vi "콜라 자판기.vi"() -> ()   [LabVIEW 2018]
panel:
  out "링":u16(ring)
  in  "종료":bool
  in  "반환":bool
  in  "구매":bool
  out "투입 금액":dbl
  in  "동전":cluster{bool, bool, bool, bool}
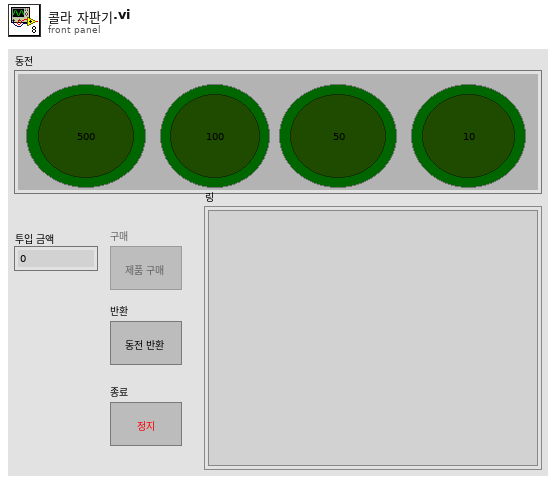
[diagram p1: front panel]
types:
  T1 = enum8{"Enabled", "Disabled", "Disabled and Grayed Out"}
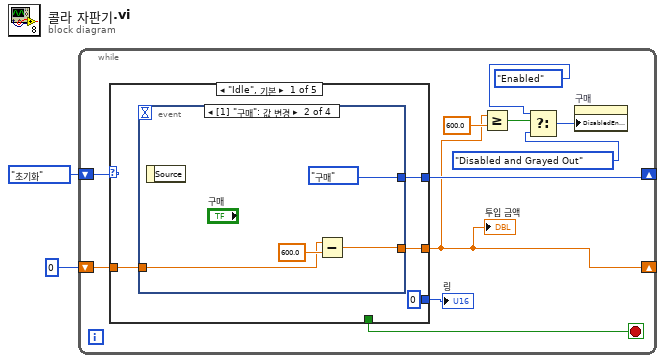
[diagram p0: block diagram]
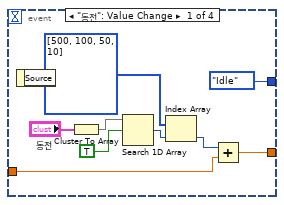
[diagram p2: hidden frame]
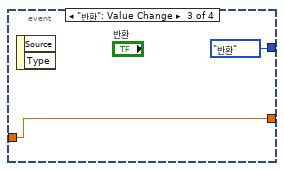
[diagram p3: hidden frame]
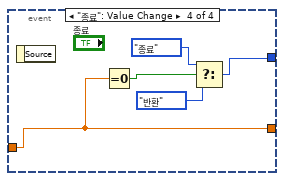
[diagram p4: hidden frame]
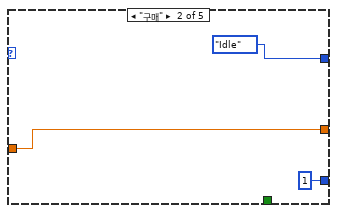
[diagram p5: hidden frame]
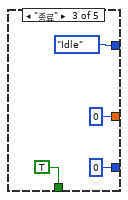
[diagram p6: hidden frame]
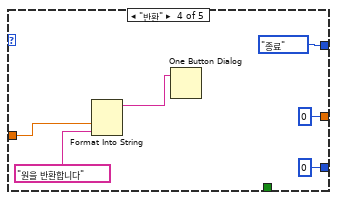
[diagram p7: hidden frame]
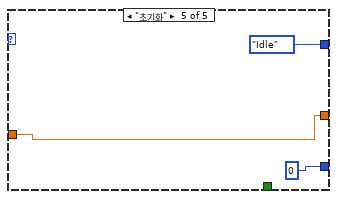
[diagram p8: hidden frame]
diagram:
  n1 = while {
    shift-right: [w12] -> _
    shift-left: enum16{"Idle", "초기화", "종료", "구매", "반환"}."초기화" ("열거형") -> [w13]
    shift-right: [w9] -> _
    shift-left: 0 -> [w11]
    stop <- w3 stop-if-true
    n2 = case shown="\"Idle\", 기본" w13 {
      tunnel: [w17 enum16{"Idle", "초기화", "종료", "구매", "반환"}."Idle" ("열거형") enum16{"Idle", "초기화", "종료", "구매", "반환"}."Idle" ("열거형") enum16{"Idle", "초기화", "종료", "구매", "반환"}."종료" ("열거형") enum16{"Idle", "초기화", "종료", "구매", "반환"}."Idle" ("열거형")] -> w12
      tunnel: [w16 w38 0 0 w53] -> w9
      tunnel: w11 -> [w15 w38 _ w47 w53]
      tunnel: [u16 0 ("링") u16 1 ("링") u16 0 ("링") u16 0 ("링") u16 0 ("링")] -> w4
      tunnel: [_ _ TRUE _ _] -> w3
      frame "Idle", Default {
        n3 = event shown="[1] \"구매\": 값 변경" {
          selector: _ -> [_ _ _ _]
          dyn-events: _ -> [_ _ _ _]
          timeout: _ -> [_ _ _ _]
          tunnel: [enum16{"Idle", "초기화", "종료", "구매", "반환"}."Idle" ("열거형") enum16{"Idle", "초기화", "종료", "구매", "반환"}."구매" ("열거형") enum16{"Idle", "초기화", "종료", "구매", "반환"}."반환" ("열거형") w35] -> w17
          tunnel: [w19 w28 w32 w37] -> w16
          tunnel: w15 -> [w18 w29 w32 w37]
          event "동전": Value Change {
            n4 = event-data() -> ()  [unwired: 1 in, 1 out]
            n5 = Cluster To Array(cluster="동전") -> (array=w24:bool[])
            n6 = Search 1D Array(1D array=w24, element=TRUE ("원소")) -> (index of element=w22:i32)  [unwired: 1 in]
            n7 = Index Array(array=i32[] [500, 100, 50, 10], index=w22) -> (element=w20:i32)
            n8 = Add(x=w20, y=w18) -> (x+y=w19:dbl)
          }
          event "구매": Value Change {
            n9 = event-data() -> ()  [unwired: 1 in, 1 out]
            n10 = Subtract(x=w29, y=600.0) -> (x-y=w28:dbl)
          }
          event "반환": Value Change {
            n11 = event-data() -> ()  [unwired: 1 in, 2 out]
          }
          event "종료": Value Change {
            n12 = event-data() -> ()  [unwired: 1 in, 1 out]
            n13 = Equal To 0?(x=w37) -> (x = 0?=w36:bool)
            n14 = Select(t=enum16{"Idle", "초기화", "종료", "구매", "반환"}."종료" ("열거형"), s=w36, f=enum16{"Idle", "초기화", "종료", "구매", "반환"}."반환" ("열거형")) -> (s? t:f=w35:enum16{"Idle", "초기화", "종료", "구매", "반환"})
          }
        }
      }
      frame "구매" {
      }
      frame "종료" {
      }
      frame "반환" {
        n15 = Format Into String(w47, "원을 반환합니다") -> (resulting string=w45:string)  [unwired: 3 in, 1 out]
        n16 = One Button Dialog(message=w45) -> ()  [unwired: 1 in, 1 out]
      }
      frame "초기화" {
      }
    }
    "투입 금액" <- w9
    "링" <- w4
    n17 = Greater Or Equal?(x=w9, y=600.0) -> (x >= y?=w8:bool)
    n18 = Select(t=T1."Enabled" ("비활성화"), s=w8, f=T1."Disabled and Grayed Out" ("비활성화")) -> (s? t:f=w7:T1)
    n19 = property on="구매" class="Bool"("DisabledEnum"=w7) -> ()  [unwired: 2 in, 2 out]
  }
